vi "Loop Frequency.vi"() -> (0 "Loop Rate (Hz)":u32)   [LabVIEW 2013, in "LVH-LINX.lvlib"]
doc: "Place this VI in a loop to calculate the loop rate. Using multiple copies of this VI in an application is not supported and will return incorrect results."
uses:
  <vilib>/LabVIEW Hacker/LINX/LVH-LINX.lvlib
  <vilib>/ptbypt/NI_PtbyPt.lvlib
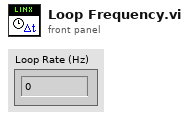
[diagram p1: front panel]
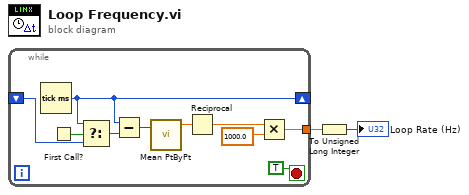
[diagram p0: block diagram]
diagram:
  n1 = while {
    shift-right: [w7] -> _
    shift-left: _ -> [w6]
    tunnel: [w3] -> w2
    stop <- TRUE stop-if-true
    n2 = Tick Count (ms)() -> (millisecond timer value=w7:u32)
    n3 = First Call?() -> (First Call?: T/F=w12:bool)
    n4 = Select(t=w7, s=w12, f=w6) -> (s? t:f=w11:u32)
    n5 = Subtract(x=w7, y=w11) -> (x-y=w10:u32)
    n6 = call <vilib>:"Mean PtByPt.vi"("x"=w10) -> ("mean"=w9:dbl)  [unwired: 3 in, 1 out]
    n7 = Reciprocal(x=w9) -> (1/x=w4:dbl)
    n8 = Multiply(x=w4, y=1000.0) -> (x*y=w3:dbl)
  }
  n9 = To Unsigned Long Integer(number=w2) -> (unsigned 32bit integer=→"Loop Rate (Hz)":u32)
